vi "GetExportFolderPath.vi"(8 "error in (no error)":errorcluster, 10 "Export Folder Name (ExportedData)":path=path "ExportedData", 11 "DisplayWaveforms":refnum<class "DisplayWaveforms.lvclass">) -> (0 "error out":errorcluster, 2 "Export File Folder":path, 3 "DisplayWaveforms out":refnum<class "DisplayWaveforms.lvclass">)   [LabVIEW 2018, in "DisplayWaveform.lvlib" / "DisplayWaveforms.lvclass"]
doc: "Get the folder path for the export"
uses:
  DisplayWaveforms.lvclass
panel:
  # "For instructions on how to use the JKI State Machine Objects, examples and video tutorials, visit:\nhttp://jki.net/state-machine-objects/\n\nJKI State Machine Objects™\nhttp://jki.net/state-machine-objects/\nCopyright (C) 2005-2015, JKI <info@jki.net>\nALL RIGHTS RESERVED"
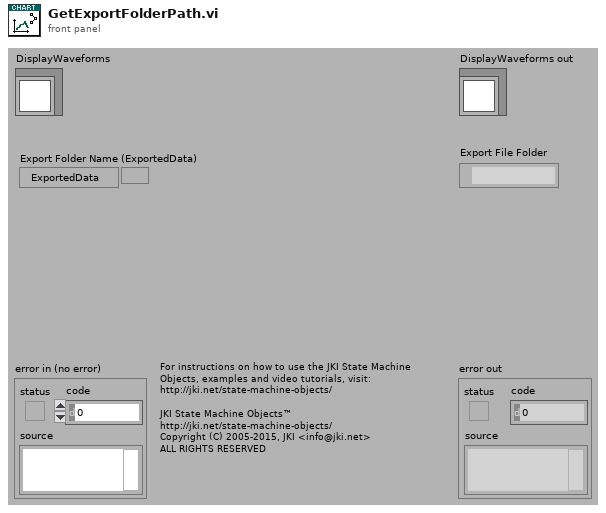
[diagram p1: front panel]
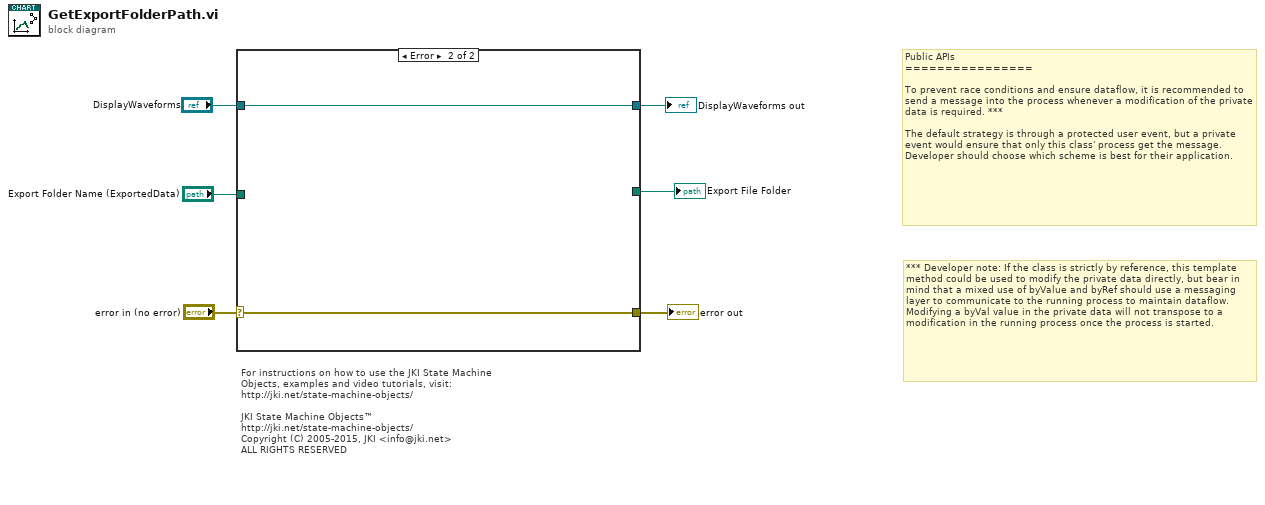
[diagram p0: block diagram]
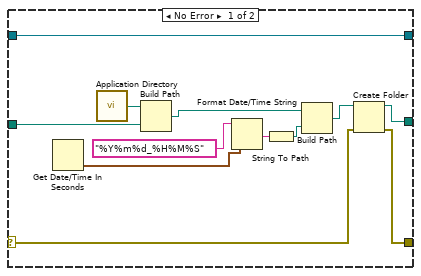
[diagram p2: hidden frame]
diagram:
  # "*** Developer note: If the class is strictly by reference, this template method could be used to modify the private data directly, but bear in mind that a mixed use of byValue and byRef should use a messaging layer to communicate to the running process to maintain dataflow. Modifying a byVal value in the private data will not transpose to a modification in the running process once the process is started."
  # "Public APIs\n================\n\nTo prevent race conditions and ensure dataflow, it is recommended to send a message into the process whenever a modification of the private data is required. ***\n\nThe default strategy is through a protected user event, but a private event would ensure that only this class' process get the message. Developer should choose which scheme is best for their application."
  # "For instructions on how to use the JKI State Machine Objects, examples and video tutorials, visit:\nhttp://jki.net/state-machine-objects/\n\nJKI State Machine Objects™\nhttp://jki.net/state-machine-objects/\nCopyright (C) 2005-2015, JKI <info@jki.net>\nALL RIGHTS RESERVED"
  n1 = case shown="Error" "error in (no error)" {
    selector: "error in (no error)" -> [w9 w19]
    tunnel: "DisplayWaveforms" -> [w7 w20]
    tunnel: [w8 w19] -> w5
    tunnel: [w7 w20] -> w4
    tunnel: "Export Folder Name (ExportedData)" -> [w11 _]
    tunnel: [w10 _] -> w1
    frame No Error {
      n2 = Get Date/Time In Seconds() -> (seconds since 1Jan1904=w17:timestamp)
      n3 = call <vilib>:"Application Directory.vi"() -> ("Application Directory"=w18:path)
      n4 = Build Path(base path=w18, name or relative path=w11) -> (appended path=w15:path)
      n5 = Format Date/Time String(time format string (%c)="%Y%m%d_%H%M%S", seconds (now)=w17) -> (date/time string=w13:string)  [unwired: 1 in]
      n6 = String To Path(string=w13) -> (path=w14:path)
      n7 = Build Path(base path=w15, name or relative path=w14) -> (appended path=w12:path)
      n8 = Create Folder(path (use dialog)=w12, error in=w9) -> (created path=w10:path, error out=w8:errorcluster)  [unwired: 1 in, 1 out]
    }
    frame Error {
    }
  }
  "error out" <- w5
  "DisplayWaveforms out" <- w4
  "Export File Folder" <- w1
